vi "TEST_L0_SUM_(1ST).vi"(4 "Voltages comprobation":dbl[](array[numeric])=[0.05, 0.1, 0.2, 0.5, 0.8], 5 "Serial number":string="SN018", 6 "IB_Clip":i32[](array[numeric])=[7, 23, 31, 63], 7 "Save NOW!":bool, 8 "error in":errorcluster, 9 "Cycles Burst":i32=10000, 10 "Channels":i32[](array[numeric])=[0, 1, 2, 3, 4, 5, 6], 11 "Instrument VISA in":T1={"AWG VISA"="generadorpulsos", "Oscilloscope  VISA "="Oscilloscope", "Integration Board IP"="172.16.7.43", "connection ID"=refnum, "report out"=refnum, "report file path"=path "C:/Documents and Settings/CTA_LAB01/Desktop/L0_Asic/L0 Asic Test Data"}) -> (0 "error out":errorcluster, 3 "Instrument VISA out":T1={"AWG VISA"="generadorpulsos", "Oscilloscope  VISA "="Oscilloscope", "Integration Board IP"="172.16.7.43", "connection ID"=refnum, "report out"=refnum, "report file path"=path "C:/Documents and Settings/CTA_LAB01/Desktop/L0_Asic/L0 Asic Test Data"})   [LabVIEW 2009]
uses:
  <vilib>/Utility/NIReport.llb/NI_report.lvclass
  <vilib>/Utility/NIReport.llb/HTML/NI_HTML.lvclass
  Sum_Abrilader/L0_Sum_Adder Folder/C/Program Files/National Instruments/LabVIEW 2012/instr.lib/Agilent 8000 Series/Public/Configure/Configure Math (Binary Operation).vi
  <instrlib>/Agilent 8000 Series/Public/Data/Read (Multiple Waveforms).vi
  Sum_Abrilader/L0_Sum_Adder Folder/C/Program Files/National Instruments/LabVIEW 2012/instr.lib/Agilent 81150/Agilent 81150.lvlib
  Sum_Abrilader/L0_Sum_Adder Folder/C/Program Files/National Instruments/LabVIEW 2012/instr.lib/Agilent 8000 Series/Agilent 8000 Series.lvlib
panel:
  out "ClipRect":dbl=136149.0
  in  "Atenuation":i32[](array[numeric])=[0, 15]
  out "dt":dbl=3.125e-12
  out "report file path":path=path "C:/Documents and Settings/CTA_LAB01/Desktop/L0_Asic/L0 Asic Test Data"
  in  "Full waveform":bool
  out "Waveform Data":waveform(dbl)[](graph)=[{"t0"=timestamp(-6.010937525502413e-09 s since 1904-01-01), "dt"=3.125e-12, "Y"=array[6408 elements]}, {"t0"=timestamp(-6.010937525502413e-09 s since 1904-01-01), "dt"=3.125e-12, "Y"=array[6408 elements]}]
  out "time for channel bucle":u32=4294966675
  out "iindex inner bucle":u16=109
  out "time attenuation bucle":u32=136149
  out "points quantity":dbl=15.0
  out "appended array":dbl[](array[numeric])=[9.99999e+37, 9.99999e+37, 2.137332e-09, 7.2166e-11, 9.99999e+37, 9.99999e+37, 9.99999e+37, 9.99999e+37, 9.99999e+37, 9.99999e+37, 15.0]
  out "read buffer 3":string="V amptd(1),9.99999E+37,9.99999E+37,9.99999E+37,9.99999E+37,9.99999E+37,1.5E+01,+ width(1),2.18163E-09,2.01279E-09,2.26658E-09,2.137332E-09,7.2166E-11,1.5E+01,V amptd(f2),9.99999E+37,9.99999E+37,9.99999E+37,9.99999E+37,9.99999E+37,1.5E+01,+ width(f2),9.99999E+37,9.99999E+37,9.99999E+37,9.99999E+37,9.99999E+37,9E+00,Time(1-f2),9.99999E+37,9.99999E+37,9.99999E+37,9.99999E+37,9.99999E+37,1.3E+01\n"
  out "bucle for inner bucle":u32=363
  out "Numeric":i32=9300975
  in  "Clip_sel_b":u32
  in  "Att gain":u32=4095
  in  "Quantity of measurements":u32=50
  in  "End 2":bool
  out "Data output":dbl[][](array[numeric])=[[0.05, 0.0, 15.0, 7.0, 1.0, 9.99999e+37, 9.99999e+37, 2.14249e-09, 8.3497e-11, 9.99999e+37, 9.99999e+37, 9.99999e+37, 9.99999e+37, 9.99999e+37, 9.99999e+37, 17.0, 0.0336, -0.00019404761904761897, 105.0], [0.05, 0.0, 15.0, 31.0, 1.0, 9.99999e+37, 9.99999e+37, 2.188109e-09, 8.187e-11, 9.99999e+37, 9.99999e+37, 9.99999e+37, 9.99999e+37, 9.99999e+37, 9.99999e+37, 14.0, 0.0336, -0.00019404761904761897, 106.0], [0.05, 0.0, 15.0, 63.0, 1.0, 9.99999e+37, 9.99999e+37, 2.133683e-09, 8.8016e-11, 9.99999e+37, 9.99999e+37, 9.99999e+37, 9.99999e+37, 9.99999e+37, 9.99999e+37, 15.0, 0.0336, -0.00019404761904761897, 107.0], [0.05, 1.0, 15.0, 7.0, 1.0, 9.99999e+37, 9.99999e+37, 2.137332e-09, 7.2166e-11, 9.99999e+37, 9.99999e+37, 9.99999e+37, 9.99999e+37, 9.99999e+37, 9.99999e+37, 15.0, 0.0336, -0.00019404761904761897, 108.0]]
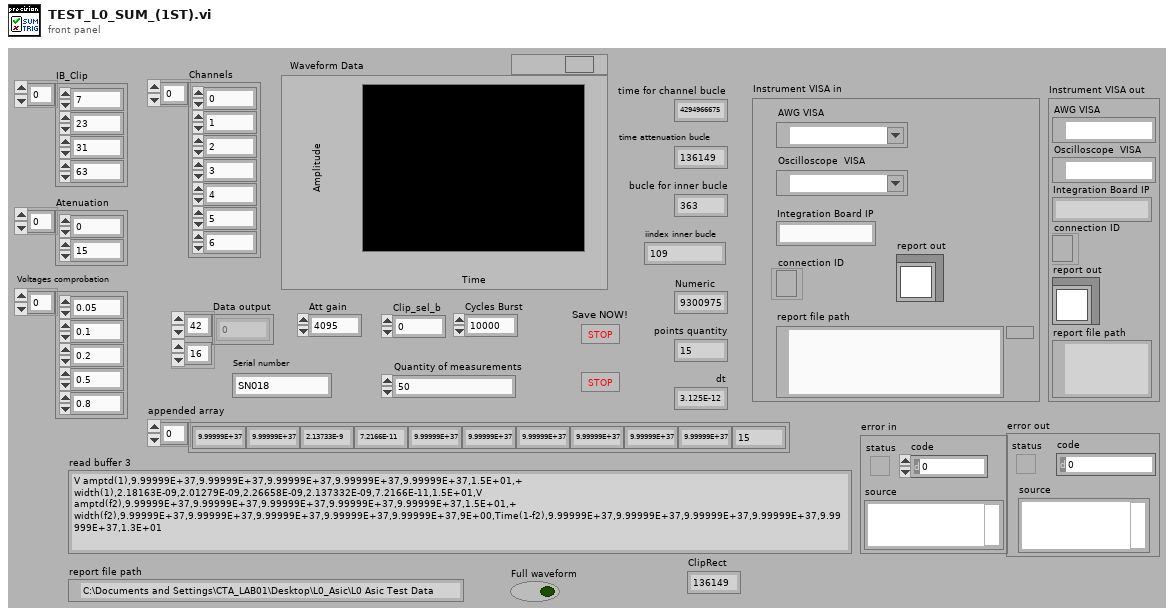
[diagram p1: front panel]
types:
  T1 = cluster{"AWG VISA":refnum<visa-resource-name>, "Oscilloscope  VISA ":refnum<visa-resource-name>, "Integration Board IP":string, "connection ID":refnum<k5>, "report out":refnum<class "NI_report.lvclass">, "report file path":path}
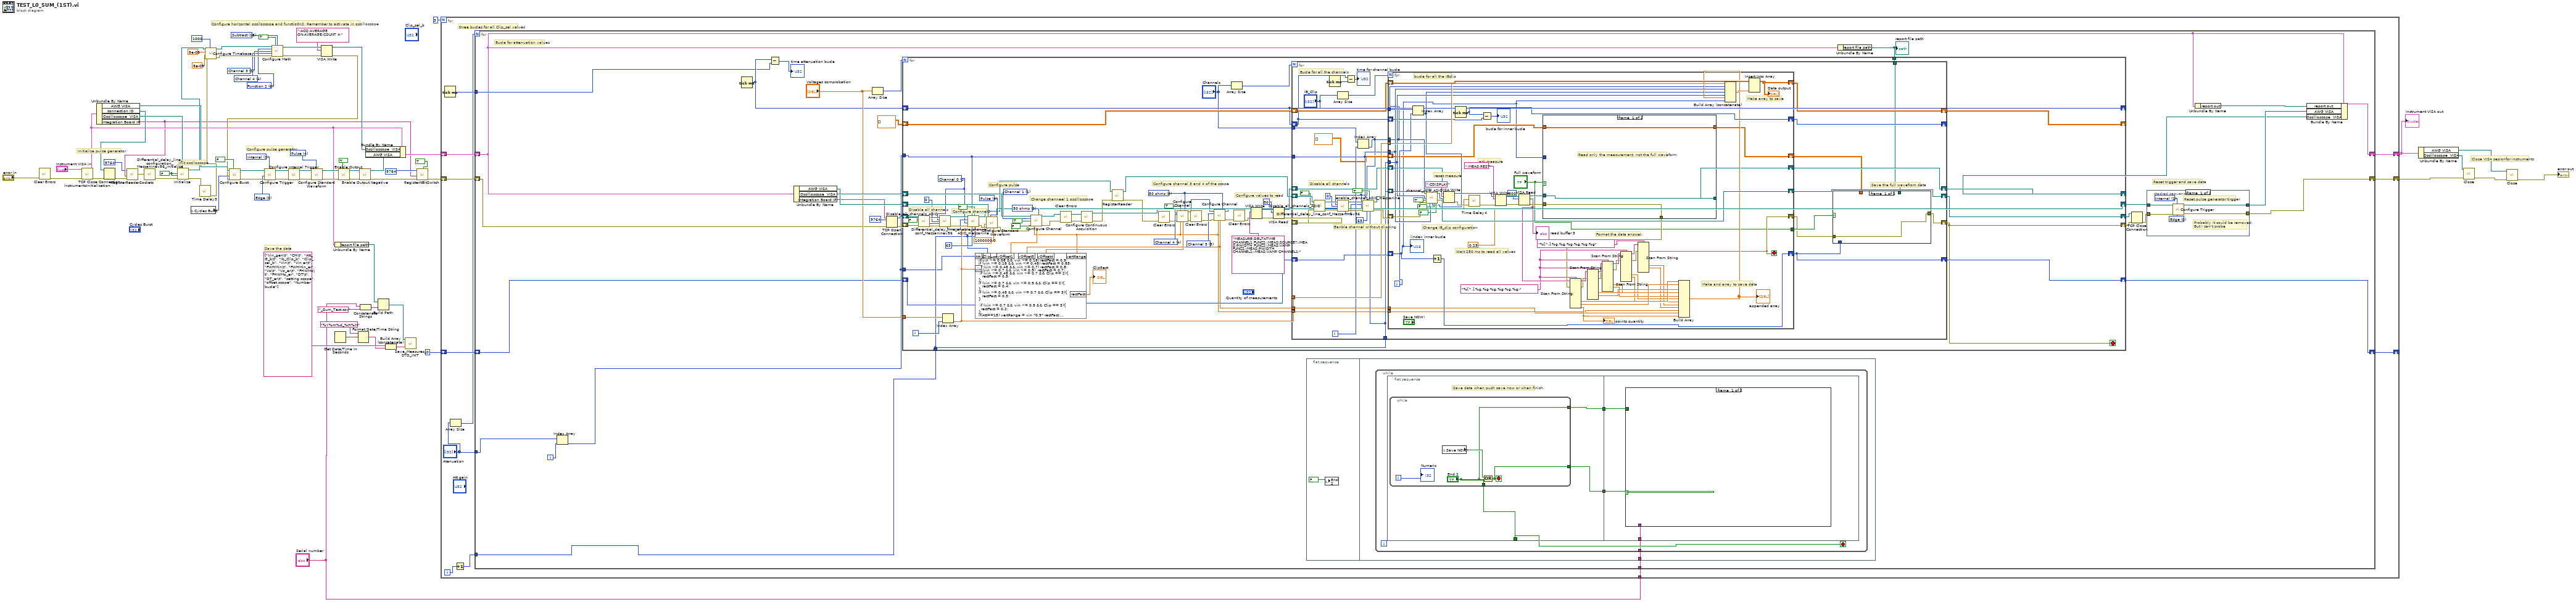
[diagram p0: block diagram]
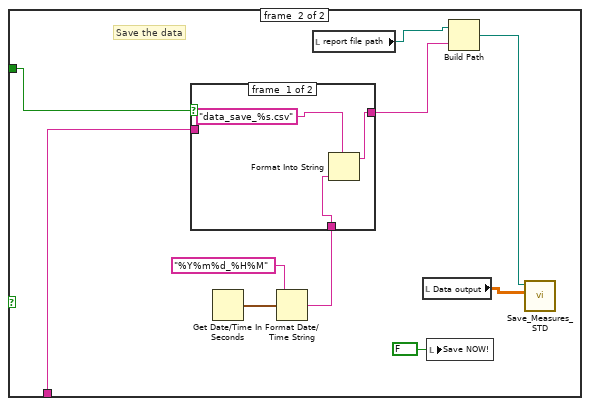
[diagram p2: hidden frame]
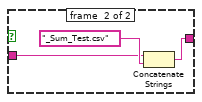
[diagram p3: hidden frame]
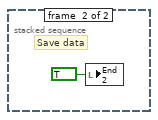
[diagram p4: hidden frame]
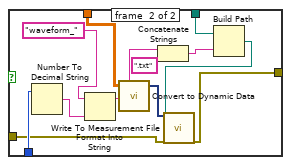
[diagram p5: hidden frame]
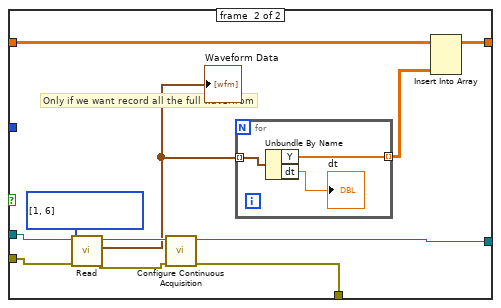
[diagram p6: hidden frame]
diagram:
  w44 = u16 6 items=["Function 1"=5, "Function 2"=6, "Function 3"=7, "Function 4"=8] ("Math Channel (5: Function 1)")
  w48 = u16 15 items=["Add"=12, "Divide"=13, "Multiply"=14, "Subtract"=15, "Common Mode"=16, "Versus"=17] ("Math Operation (12: Add)")
  w43 = 3 items=["Channel 1"=1, "Channel 2"=2, "Channel 3"=3, "Channel 4"=4] ("Channel (1: Channel 1)")
  w42 = 4 items=["Channel 1"=1, "Channel 2"=2, "Channel 3"=3, "Channel 4"=4] ("Channel (1: Channel 1)")
  w63 = u16 1 items=["Immediate", "Internal", "External", "Software Trigger Function"] ("Trigger Source (0: Immediate)")
  w64 = u16 0 items=["Edge", "Level"] ("Trigger Mode (0: Edge)")
  w68 = u16 4 items=["Sine", "Square", "Ramp Up", "Ramp Down", "Pulse", "Noise", "DC"] ("Waveform (0: Sine)")
  w72 = FALSE ("ID Query (True)")
  # "Save the data"
  # "Configure horizontal osciloscope and functio0n2. Remember to activate in oscilloscope"
  # "Close VISA sesionfor instruments"
  # "Configure pulse generator"
  # "Init osciloscope"
  # "Initialize pulse generator"
  n1 = call <vilib>:"Clear Errors.vi"("error in (no error)"="error in") -> ("error out"=w70:errorcluster)  [unwired: 6 in]
  n2 = call "instrumentsInitialization.vi"("error in"=w70, "Instrument VISA in"="Instrument VISA in") -> ("error out"=w11:errorcluster, "Instrument VISA out"=w19:T1)  [unwired: 8 in]
  n3 = Unbundle By Name(w19) -> ("AWG VISA"=w54:refnum<visa-resource-name>, "connection ID"=w58:refnum<k5>, "Oscilloscope  VISA"=w55:refnum<visa-resource-name>, "Integration Board IP"=w3:string)
  n4 = TCP Close Connection(connection ID=w58, error in (no error)=w11) -> (error out=w4:errorcluster)  [unwired: 1 in, 1 out]
  n5 = call "RegisterReaderSockets.vi"("error in (no error)"=w4, "IP"=w3, "Port"=u16 9764 ("remote port or service name")) -> ("error out"=w1:errorcluster)  [unwired: 7 in]
  n6 = call "Differential_delay_line_configuration_Mezzaninev56_initialize.vi"("error in (no error)"=w1) -> ("error out 2"=w10:errorcluster)  [unwired: 1 in]
  n7 = call "Initialize.vi"("error in (no error)"=w10, "Reset (True)"=w72, "ID Query (True)"=w72, "VISA resource name"=w55) -> ("error out"=w71:errorcluster, "VISA resource name out"=w41:refnum<visa-resource-name>)  [unwired: 6 in]
  n8 = local read "Cycles Burst"() -> (w67:i32)
  n9 = call "Time Delay3"("error in (no error)"=w71) -> ("error out"=w40:errorcluster)  [unwired: 10 in]
  n10 = call "Configure Timebase.vi"("Record Length (1000)"=1000, "error in (no error)"=w40, "Position (0.0 s)"=8e-09, "Timebase (0.005 s)"=5e-08, "VISA resource name"=w41) -> ("error out"=w45:errorcluster, "VISA resource name out"=w46:refnum<visa-resource-name>)  [unwired: 5 in]
  n11 = call-poly "Configure Math.vi"("VISA resource name"=w46, "Enable Math Channel (T:Enable)"=TRUE, "Math Operation (12: Add)"=w48, "Math Channel (5: Function 1)"=w44, "Math Operand (1: Channel 1)"=w43, "Math Operand (2: Channel 2)"=w42, "error in (no error)"=w45) -> ("VISA resource name out"=w16:refnum<visa-resource-name>, "error out"=w15:errorcluster)  [unwired: 7 in]
  n12 = VISA Write(VISA resource name=w16, write buffer=":ACQ:AVERAGE ON;AVERAGE:COUNT 4;", error in (no error)=w15) -> (VISA resource name out=w13:refnum<visa-resource-name>, error out=w14:errorcluster)  [unwired: 1 out]
  n13 = call "Configure Burst.vi"("Enable Burst (F: Disable)"=FALSE, "error in (no error)"=w14, "Burst Count (2)"=w67, "VISA resource name"=w54) -> ("error out"=w66:errorcluster, "VISA resource name out"=w65:refnum<visa-resource-name>)  [unwired: 6 in]
  n14 = call "Configure Trigger.vi"("Trigger Source (0: Immediate)"=w63, "error in (no error)"=w66, "Trigger Mode (0: Edge)"=w64, "VISA resource name"=w65) -> ("error out"=w62:errorcluster, "VISA resource name out"=w61:refnum<visa-resource-name>)  [unwired: 6 in]
  n15 = call "Configure Internal Trigger.vi"("error in (no error)"=w62, "VISA resource name"=w61) -> ("error out"=w59:errorcluster, "VISA resource name out"=w60:refnum<visa-resource-name>)  [unwired: 8 in]
  n16 = call "Configure Standard Waveform.vi"("Waveform (0: Sine)"=w68, "error in (no error)"=w59, "VISA resource name"=w60) -> ("error out"=w53:errorcluster, "VISA resource name out"=w52:refnum<visa-resource-name>)  [unwired: 7 in]
  n17 = Unbundle By Name(w19) -> ("report file path"=w20:path)
  n18 = Get Date/Time In Seconds() -> (seconds since 1Jan1904=w25:timestamp)
  n19 = call "Enable Output.vi"("Enable Output (T: Enable)"=TRUE, "error in (no error)"=w53, "VISA resource name"=w52) -> ("error out"=w31:errorcluster, "VISA resource name out"=w30:refnum<visa-resource-name>)  [unwired: 7 in]
  n20 = Format Date/Time String(time format string (%c)="%Y%m%d_%H%M", seconds (now)=w25) -> (date/time string=w23:string)  [unwired: 1 in]
  n21 = call "Enable Output Negative.vi"("error in (no error)"=w31, "VISA resource name"=w30) -> ("error out"=w9:errorcluster, "VISA resource name out"=w29:refnum<visa-resource-name>)  [unwired: 8 in]
  n22 = Concatenate Strings("Serial number", "_Sum_Test.csv" ("format string")) -> (w21:string)
  n23 = Bundle By Name(cluster=w19, "Oscilloscope  VISA"=w13, "AWG VISA"=w29) -> (w7:T1)
  n24 = Build Path(base path=w20, name or relative path=w21) -> (appended path=w28:path)
  n25 = Build Array (concatenate)(string[] ["Vin_gen\t", "CH\t", "Att_G_b\t", "Ib_Clip_b", "Clip_sel_b", "Vin\t", "Vin er\t", "FWHMin\t", "FWHMin_er", "Vo\t", "Vo_er\t", "FHWMo\t", "FHWMo_er", "DT\t", "DT_er\t", "setting scope", "offset scope", "Number bucle"] ("appended array"), w23) -> (w26:string[])
  n26 = call "Save_Measures_STD_INIT.vi"("appended array"=w26, "file path (dialog if empty)"=w28) -> ()  [unwired: 10 in]
  n27 = call "RegisterNBitSwitch.vi"("Switch Bit"=TRUE ("Enable Output (T: Enable)"), "error in (no error)"=w9, "IP"=w3, "Port"=u16 9764 ("remote port or service name")) -> ("error out"=w8:errorcluster)  [unwired: 7 in]
  n28 = for {
    N: 3 -> [_]
    shift-right: [w84] -> w35
    shift-left: w8 -> [w80]
    shift-right: [w83] -> w18
    shift-left: w7 -> [w79]
    shift-right: [w76] -> _
    shift-left: u16 0 ("remote port or service name") -> [w77]
    tunnel: "Serial number" -> [w73]
    i -> [w81]
    # "three bucles for all Clip_sel values"
    n29 = Tick Count (ms)() -> (millisecond timer value=w78:u32)
    n30 = Array Size(array="Atenuation") -> (size(s)=w75:i32)
    n31 = Increment(x=w81) -> (x+1=w82:i32)
    n32 = for {
      N: w75 -> [_]
      shift-right: [w89] -> w84
      shift-left: w80 -> [w106]
      shift-right: [w113] -> w83
      shift-left: w79 -> [w93]
      tunnel: w82 -> [w91]
      tunnel: w78 -> [w98]
      shift-right: [w96] -> w76
      shift-left: w77 -> [w97]
      tunnel: "Atenuation" -> [w87]
      tunnel: w73 -> [w86]
      i -> [w88]
      # "Reset trigger and save data"
      # "Bucle for attenuation values"
      n33 = Index Array(array=w87, index=w88) -> (element=w85:i32)
      n34 = Tick Count (ms)() -> (millisecond timer value=w99:u32)
      n35 = Subtract(x=w99, y=w98) -> (x-y=→"time attenuation bucle":u32)
      n36 = Unbundle By Name(w93) -> ("AWG VISA"=w110:refnum<visa-resource-name>, "Oscilloscope  VISA"=w111:refnum<visa-resource-name>, "Integration Board IP"=w107:string)
      n37 = Array Size(array="Voltages comprobation") -> (size(s)=w114:i32)
      n38 = TCP Open Connection(address=w107, remote port or service name=u16 9764, error in (no error)=w106) -> (connection ID=w101:refnum<k5>, error out=w105:errorcluster)  [unwired: 2 in]
      n39 = flat-sequence {
        tunnel: w86 -> [w117]
        frame #0 {
          n40 = local write "End 2"(FALSE ("End")) -> ()
        }
        frame #1 {
          n41 = while {
            tunnel: w117 -> [w118]
            stop <- w119 stop-if-true
            n42 = flat-sequence {
              tunnel: [w124] -> w121
              tunnel: [w123] -> w120
              tunnel: [w122] -> w119
              tunnel: w121 -> [w131]
              tunnel: w120 -> [w130]
              tunnel: w118 -> [w129]
              frame #0 {
                # "Save data when push save now or when finish."
                n43 = while {
                  tunnel: [w127] -> w124
                  tunnel: ["End 2"] -> w123
                  tunnel: ["End 2"] -> w122
                  i -> [w126]
                  stop <- w127 stop-if-true
                  n44 = local read "Save NOW!"() -> (w128:bool)
                  n45 = Or(x=w128, y="End 2") -> (x .or. y?=w127:bool)
                  "Numeric" <- w126
                }
              }
              frame #1 {
                n46 = case shown="True" w131 {
                  tunnel: w130 -> [_ w138]
                  tunnel: w129 -> [_ w132]
                  frame #0 {
                  }
                  frame #1 {
                    # "Save the data"
                    n47 = Get Date/Time In Seconds() -> (seconds since 1Jan1904=w135:timestamp)
                    n48 = Format Date/Time String(time format string (%c)="%Y%m%d_%H%M", seconds (now)=w135) -> (date/time string=w133:string)  [unwired: 1 in]
                    n49 = case shown="True" w138 {
                      tunnel: [w143 w145] -> w137
                      tunnel: w133 -> [w142 _]
                      tunnel: w132 -> [_ w146]
                      frame #0 {
                        n50 = Format Into String(format string="data_save_%s.csv", w142) -> (resulting string=w143:string)  [unwired: 2 in, 1 out]
                      }
                      frame #1 {
                        n51 = Concatenate Strings(w146, "_Sum_Test.csv" ("format string")) -> (w145:string)
                      }
                    }
                    n52 = local read "report file path"() -> (w136:path)
                    n53 = local read "Data output"() -> (w140:dbl[][])
                    n54 = local write "Save NOW!"(FALSE ("Save NOW!")) -> ()
                    n55 = Build Path(base path=w136, name or relative path=w137) -> (appended path=w141:path)
                    n56 = call "Save_Measures_STD.vi"("Data in"=w140, "file path (dialog if empty)"=w141) -> ()  [unwired: 10 in]
                  }
                }
              }
            }
          }
        }
      }
      n57 = Unbundle By Name(w93) -> ("report file path"=w92:path)
      "report file path" <- w92
      n58 = for {
        N: w114 -> [_]
        shift-right: [w159] -> w103
        shift-left: w105 -> [w203]
        shift-right: [w216] -> _
        shift-left: dbl[][] [] -> [w217]
        tunnel: "Voltages comprobation" -> [w215]
        shift-right: [w195] -> w112
        shift-left: w110 -> [w223]
        shift-right: [w212] -> w94
        shift-left: w111 -> [w208]
        tunnel: w85 -> [w210]
        tunnel: w91 -> [w173]
        shift-right: [w160] -> w102
        shift-left: w101 -> [w202]
        shift-right: [w180] -> _
        shift-left: w99 -> [w180]
        shift-right: [w179] -> w96
        shift-left: w97 -> [w191]
        tunnel: w92 -> [w178]
        tunnel: w85 -> [w172]
        i -> [w222]
        stop <- w159 stop-if-true
        w184 = 3 items=["Channel 1"=1, "Channel 2"=2, "Channel 3"=3, "Channel 4"=4] ("Channel (1: Channel 1)")
        w204 = 4 items=["Channel 1"=1, "Channel 2"=2, "Channel 3"=3, "Channel 4"=4] ("Channel (1: Channel 1)")
        w185 = u32 0 items=["50 ohms", "1 Mohms"] ("Input Impedance (1: 1 Mohms)")
        w162 = u16 0 items=["Channel 0", "Channel 1", "Channel 2", "Channel 3", "Channel 4", "Channel 5", "Channel 6"] ("Channel")
        w219 = u32 0 items=["50 ohms", "1 Mohms"] ("Input Impedance (1: 1 Mohms)")
        w221 = 1 items=["Channel 1"=1, "Channel 2"=2, "Channel 3"=3, "Channel 4"=4] ("Channel (1: Channel 1)")
        w224 = u16 4 items=["Sine", "Square", "Ramp Up", "Ramp Down", "Pulse", "Noise", "DC"] ("Waveform (0: Sine)")
        # "Configure values to read"
        # "Configure channel 3 and 4 of the scope"
        # "Change channeel 1 oscilloscope"
        # "Configure pulse"
        # "Configure channel0"
        # "Disable all channels"
        n59 = call "Disable_all_channels_ASIC.vi"("error in"=w203, "Clip_en_b"=FALSE, "connection ID"=w202) -> ("error out"=w168:errorcluster, "id_out"=w163:i32, "connection ID out"=w164:refnum<k5>)  [unwired: 6 in]
        n60 = call "Differential_delay_line_conf_Mezzaninev56.vi"("connection ID"=w164, "channel"=w162, "Delay value"=u16 0, "Id in"=w163, "error in (no error)"=w168) -> ("connection ID out"=w165:refnum<k5>, "Id out"=w166:i32, "error out 2"=w167:errorcluster)  [unwired: 3 in, 5 out]
        n61 = Index Array(array=w215, index=w222) -> (element=w174:dbl)
        n62 = call "enable_channel_ASIC_mezzanine.vi"("Clip_sel_b"=w173, "maj/sum"=TRUE, "Ib_clipVb"=u32 63, "Att gain"=w210, "error in"=w167, "Channel"=w162, "id_in"=w166, "connection ID"=w165) -> ("error out"=w211:errorcluster, "connection ID out"=w156:refnum<k5>)  [unwired: 1 in, 1 out]
        n63 = formula code="float rectFact = 1;\nif(vin >= 0.08 && vin <= 0.18) rectFact = 0.9;\nif (vin >= 0.18 && vin <= 0.48) rectFact = 0.85;\n if (vin >= 0.48 && vin <= 0.7) rectFact = 0.8;\nif (vin >= 0.7 && vin <= 0.9)  rectFact = 0.7;\n if (vin >= 0.48 && vin <= 0.7 && Clip == 2){\n   rectFact = 0.5;\n}\nif (vin >= 0.7 && vin <= 0.9 && Clip == 2){\n   rectFact = 0.4;\n}\nif (vin >= 0.48 && vin <= 0.7 && Clip == 3){\n   rectFact = 0.3;\n}\n\n if (vin >= 0.7 && vin <= 0.9 && Clip == 3){\n  rectFact = 0.2;\n}\nif(Att==15) vertRange = vin *0.9* rectFact;\nelse vertRange = vin * 1.0* rectFact;\nvOffset1  = vertRange /6;\nvOffset3  = vertRange /6;\nvOffset4  = -vertRange/6;"("vin"=w174, "Att"=w172, "Clip"=w173) -> ("vOffset1"=w176:dbl, "vOffset3"=w169:dbl, "vOffset4"=w175:dbl, "vertRange"=w170:dbl, "rectFact"=→"ClipRect":dbl)
        n64 = call "Configure Standard Waveform.vi"("Frequency (1000.0 Hz)"=1000000.0, "Waveform (0: Sine)"=w224, "error in (no error)"=w211, "Amplitude (1.0 Vpp)"=w174, "VISA resource name"=w223) -> ("error out"=w209:errorcluster, "VISA resource name out"=w195:refnum<visa-resource-name>)  [unwired: 5 in]
        n65 = call "Configure Channel.vi"("VISA resource name"=w208, "Enable Channel (Enable)"=TRUE, "BW Limit 20MHz (Disable)"=FALSE, "Input Impedance (1: 1 Mohms)"=w219, "Channel (1: Channel 1)"=w221, "error in (no error)"=w209, "Vertical Range (2.0 V)"=w170, "Vertical Offset (0.0 V)"=w176) -> ("VISA resource name out"=w207:refnum<visa-resource-name>, "error out"=w206:errorcluster)  [unwired: 6 in]
        n66 = call <vilib>:"Clear Errors.vi"("error in (no error)"=w206) -> ("error out"=w205:errorcluster)  [unwired: 6 in]
        n67 = call "Configure Continuous Acquisition.vi"("error in (no error)"=w205, "VISA resource name"=w207) -> ("error out"=w158:errorcluster, "VISA resource name out"=w177:refnum<visa-resource-name>)  [unwired: 8 in]
        n68 = call "RegisterReader.vi"("error in (no error)"=w158, "connection ID"=w156) -> ("error out"=w157:errorcluster, "connection ID out"=w155:refnum<k5>)  [unwired: 7 in]
        n69 = call <vilib>:"Clear Errors.vi"("error in (no error)"=w157) -> ("error out"=w213:errorcluster)  [unwired: 6 in]
        n70 = call "Configure Channel.vi"("VISA resource name"=w177, "Enable Channel (Enable)"=TRUE, "Input Impedance (1: 1 Mohms)"=w185, "Channel (1: Channel 1)"=w204, "error in (no error)"=w213, "Vertical Range (2.0 V)"=w170, "Vertical Offset (0.0 V)"=w175) -> ("VISA resource name out"=w187:refnum<visa-resource-name>, "error out"=w214:errorcluster)  [unwired: 7 in]
        n71 = call <vilib>:"Clear Errors.vi"("error in (no error)"=w214) -> ("error out"=w189:errorcluster)  [unwired: 6 in]
        n72 = call "Configure Channel.vi"("VISA resource name"=w187, "Input Impedance (1: 1 Mohms)"=w185, "Channel (1: Channel 1)"=w184, "error in (no error)"=w189, "Vertical Range (2.0 V)"=w170, "Vertical Offset (0.0 V)"=w169) -> ("VISA resource name out"=w186:refnum<visa-resource-name>, "error out"=w190:errorcluster)  [unwired: 8 in]
        n73 = Array Size(array="Channels") -> (size(s)=w196:i32)
        n74 = call <vilib>:"Clear Errors.vi"("error in (no error)"=w190) -> ("error out"=w188:errorcluster)  [unwired: 6 in]
        n75 = VISA Write(VISA resource name=w186, write buffer="MEASURE:DELTATIME CHANNEL1,FUNC2;:MEAS:SOURCE?;:MEAS:PWIDTH FUNC2;:MEAS:VAMP FUNC2;:MEAS:PWIDTH CHANNEL1;:MEAS:VAMP CHANNEL1;", error in (no error)=w188) -> (VISA resource name out=w201:refnum<visa-resource-name>, error out=w200:errorcluster)  [unwired: 1 out]
        n76 = VISA Read(VISA resource name=w201, byte count=u32 50, error in (no error)=w200) -> (VISA resource name out=w197:refnum<visa-resource-name>, error out=w198:errorcluster)  [unwired: 2 out]
        n77 = for {
          N: w196 -> [_]
          tunnel: w210 -> [w243]
          tunnel: w173 -> [w251]
          tunnel: w174 -> [w263]
          shift-right: [w265] -> w216
          shift-left: w217 -> [w266]
          shift-right: [w264] -> w212
          shift-left: w197 -> [w261]
          shift-right: [w262] -> w160
          shift-left: w155 -> [w255]
          shift-right: [w241] -> w159
          shift-left: w198 -> [w257]
          tunnel: "Channels" -> [w260]
          shift-right: [w237] -> w179
          shift-left: w191 -> [w258]
          shift-right: [w245] -> _
          shift-left: w180 -> [w246]
          tunnel: w178 -> [w239]
          tunnel: w170 -> [w235]
          tunnel: w169 -> [w234]
          i -> [w259]
          # "Eanble channel without clipping"
          # "Disable all channels"
          # "Save the full wavefrom data"
          # "Bucle for all the channels"
          n78 = call "Disable_all_channels_ASIC.vi"("error in"=w257, "Clip_en_b"=FALSE, "connection ID"=w255) -> ("error out"=w233:errorcluster, "id_out"=w229:i32, "connection ID out"=w231:refnum<k5>)  [unwired: 6 in]
          n79 = Tick Count (ms)() -> (millisecond timer value=w247:u32)
          n80 = Array Size(array="IB_Clip") -> (size(s)=w249:i32)
          n81 = Subtract(x=w246, y=w247) -> (x-y=→"time for channel bucle":u32)
          n82 = Index Array(array=w260, index=w259) -> (element=w228:i32)
          n83 = call "Differential_delay_line_conf_Mezzaninev56.vi"("connection ID"=w231, "channel"=w228, "Delay value"=u16 0, "Id in"=w229, "error in (no error)"=w233) -> ("connection ID out"=w230:refnum<k5>, "Id out"=w227:i32, "error out 2"=w232:errorcluster)  [unwired: 3 in, 5 out]
          n84 = call "enable_channel_ASIC_mezzanine.vi"("Clip_sel_b"=w251, "maj/sum"=TRUE, "Ib_clipVb"=u32 63, "Att gain"=w243, "error in"=w232, "Channel"=w228, "id_in"=w227, "connection ID"=w230) -> ("error out"=w256:errorcluster, "connection ID out"=w254:refnum<k5>)  [unwired: 1 in, 1 out]
          n85 = for {
            N: w249 -> [_]
            shift-right: [w289] -> w240
            shift-left: w256 -> [w313]
            tunnel: w263 -> [w344]
            shift-right: [w326] -> w265
            shift-left: w266 -> [w342]
            tunnel: w243 -> [w339]
            shift-right: [w291] -> w264
            shift-left: w261 -> [w315]
            tunnel: w251 -> [w338]
            shift-right: [w340] -> w262
            shift-left: w254 -> [w341]
            shift-right: [w335] -> w245
            shift-left: w246 -> [w336]
            tunnel: w228 -> [w298]
            shift-right: [w297] -> w237
            shift-left: w258 -> [w284]
            tunnel: "IB_Clip" -> [w296]
            shift-right: [w287] -> w238
            shift-left: dbl[][] [] ("Y") -> [w288]
            tunnel: ["Full waveform"] -> w242
            tunnel: w235 -> [w282]
            tunnel: w234 -> [w281]
            i -> [w295]
            stop <- w289 stop-if-true
            w308 = "%[^,],%g,%g,%g,%g,%g,%g," ("format string")
            # "Make and array to save data"
            # "Wait 250 ms to read all values"
            # "Change IB_clip configuration"
            # "Make array to save"
            # "Format the data answer."
            # "ask measure"
            # "reset measure"
            # "bucle for all the IBclip"
            n86 = Index Array(array=w296, index=w295) -> (element=w294:i32)
            n87 = call "channel_conf_ASIC.vi"("connection ID"=w341, "Ring"=w298, "Clip_sel_b"=w338, "CompBuf_en_b"=TRUE, "error out"=w313, "Att gain"=w339, "Ib_ClipVb"=w294, "Clip_en_b"=FALSE, "Att_en_b"=FALSE) -> ("connection ID out"=w340:refnum<k5>, "error out 2"=w311:errorcluster)  [unwired: 2 in, 3 out]
            n88 = Increment(x=w284) -> (x+1=w297:u16)
            n89 = VISA Write(VISA resource name=w315, write buffer=":CDISPLAY", error in (no error)=w311) -> (VISA resource name out=w317:refnum<visa-resource-name>, error out=w310:errorcluster)  [unwired: 1 out]
            n90 = Tick Count (ms)() -> (millisecond timer value=w335:u32)
            n91 = call "Time Delay4"("error in (no error)"=w310, "Delay Time (s)"=0.25 ("x*y")) -> ("error out"=w328:errorcluster)  [unwired: 9 in]
            n92 = Subtract(x=w335, y=w336) -> (x-y=→"bucle for inner bucle":u32)
            n93 = VISA Write(VISA resource name=w317, write buffer=":MEAS:RES?", error in (no error)=w328) -> (VISA resource name out=w333:refnum<visa-resource-name>, error out=w332:errorcluster)  [unwired: 1 out]
            n94 = VISA Read(VISA resource name=w333, byte count=u32 800, error in (no error)=w332) -> (VISA resource name out=w292:refnum<visa-resource-name>, read buffer=w329:string, error out=w293:errorcluster)  [unwired: 1 out]
            "read buffer 3" <- w329
            n95 = case shown="False" "Full waveform" {
              tunnel: w293 -> [w347 w356]
              tunnel: w292 -> [w346 w358]
              tunnel: [w346 w354] -> w291
              tunnel: [w347 w348] -> w290
              tunnel: w284 -> [_ _]
              tunnel: w288 -> [w345 w351]
              tunnel: [w345 w350] -> w287
              frame #0 {
                # "Read only the measurement, not the full waveform"
              }
              frame #1 {
                w357 = i32[] [1, 6] items=["Channel 1"=1, "Channel 2"=2, "Channel 3"=3, "Channel 4"=4, "Function 1"=5, "Function 2"=6, "Function 3"=7, "Function 4"=8, "Memory 1"=9, "Memory 2"=10, "Memory 3"=11, "Memory 4"=12] ("Channels")
                # "Only if we want record all the full waverfrom"
                n96 = call-poly <instrlib>:"Read.vi"("error in (no error)"=w356, "Channels"=w357, "VISA resource name"=w358) -> ("error out"=w353:errorcluster, "Waveform Data"=w352:waveform(dbl)[], "VISA resource name out"=w355:refnum<visa-resource-name>)  [unwired: 6 in]
                "Waveform Data" <- w352
                n97 = call "Configure Continuous Acquisition.vi"("error in (no error)"=w353, "VISA resource name"=w355) -> ("error out"=w348:errorcluster, "VISA resource name out"=w354:refnum<visa-resource-name>)  [unwired: 8 in]
                n98 = for {
                  tunnel: w352 -> [w361] mode=indexing
                  tunnel: [w360] -> w349 mode=indexing
                  n99 = Unbundle By Name(w361) -> ("Y"=w360:dbl[], "dt"=→"dt":dbl)
                }
                n100 = Insert Into Array(array=w351, new element=w349) -> (w350:dbl[][])  [unwired: 2 in]
              }
            }
            n101 = Scan From String(format string=w308, input string=w329, error in=w290) -> (remaining string=w325:string, error out=w318:errorcluster, output 5=w307:dbl, output 6=w306:dbl, output 7=w283:dbl)  [unwired: 12 in, 1 out]
            "points quantity" <- w283
            n102 = Scan From String(format string=w308, input string=w325, error in=w318) -> (remaining string=w322:string, error out=w319:errorcluster, output 5=w305:dbl, output 6=w304:dbl)  [unwired: 13 in, 1 out]
            n103 = Scan From String(format string=w308, input string=w322, error in=w319) -> (remaining string=w323:string, error out=w320:errorcluster, output 5=w280:dbl, output 6=w303:dbl)  [unwired: 13 in, 1 out]
            n104 = Scan From String(format string=w308, input string=w323, error in=w320) -> (remaining string=w324:string, error out=w321:errorcluster, output 5=w302:dbl, output 6=w301:dbl)  [unwired: 13 in, 1 out]
            n105 = Scan From String(format string="%[^,],%g,%g,%g,%g,%g,%g", input string=w324, error in=w321) -> (error out=w289:errorcluster, output 5=w300:dbl, output 6=w299:dbl)  [unwired: 13 in, 2 out]
            n106 = Build Array(w307, w306, w305, w304, w280, w303, w302, w301, w300, w299, w282, w281, w283) -> (w327:dbl[])
            "appended array" <- w327
            n107 = Build Array (concatenate)(w344, w298, w339, w294, w338, w327, w284) -> (w343:dbl[])
            n108 = Insert Into Array(array=w342, new element=w343) -> (w326:dbl[][])  [unwired: 2 in]
            "Data output" <- w326
            "iindex inner bucle" <- w284
          }
          n109 = case shown="False" w242 {
            tunnel: w238 -> [_ w279]
            tunnel: w240 -> [w267 w268]
            tunnel: [w267 w277] -> w241
            tunnel: w239 -> [_ w270]
            tunnel: w237 -> [_ w269]
            frame #0 {
            }
            frame #1 {
              n110 = Number To Decimal String(number=w269) -> (decimal integer string=w276:string)  [unwired: 1 in]
              n111 = Format Into String(initial string="waveform_", w276) -> (resulting string=w274:string)  [unwired: 2 in, 1 out]
              n112 = call "Convert to Dynamic Data"("2D Array"=w279) -> ("Dynamic Data Type"=w278:dynamicdata)  [unwired: 3 in]
              n113 = Concatenate Strings(w274, ".txt" ("string")) -> (w273:string)
              n114 = Build Path(base path=w270, name or relative path=w273) -> (appended path=w271:path)
              n115 = call "Write To Measurement File"("Signals"=w278, "error in (no error)"=w268, "Filename"=w271) -> ("error out"=w277:errorcluster)  [unwired: 14 in, 2 out]
            }
          }
        }
      }
      n116 = TCP Close Connection(connection ID=w102, error in (no error)=w103) -> (error out=w104:errorcluster)  [unwired: 1 in, 1 out]
      n117 = stacked-sequence {
        tunnel: w104 -> [w151 _]
        tunnel: [w150 _] -> w89
        tunnel: w112 -> [w149 _]
        tunnel: [w148 _] -> w95
        frame #0 {
          w152 = u16 1 items=["Immediate", "Internal", "External", "Software Trigger Function"] ("Trigger Source (0: Immediate)")
          w153 = u16 0 items=["Edge", "Level"] ("Trigger Mode (0: Edge)")
          # "Probably it could be removed. \nBut I can't probe"
          # "Reset pulse generator tirgger"
          n118 = call "Configure Trigger.vi"("Trigger Source (0: Immediate)"=w152, "error in (no error)"=w151, "Trigger Mode (0: Edge)"=w153, "VISA resource name"=w149) -> ("error out"=w150:errorcluster, "VISA resource name out"=w148:refnum<visa-resource-name>)  [unwired: 6 in]
        }
        frame #1 {
          # "Save data"
          n119 = local write "End 2"(TRUE ("End 2")) -> ()
        }
      }
      n120 = Unbundle By Name(w93) -> ("report out"=w90:refnum<class "NI_report.lvclass">)
      n121 = Bundle By Name(cluster=w93, "report out"=w90, "AWG VISA"=w95, "Oscilloscope  VISA"=w94) -> (w113:T1)
    }
  }
  "Instrument VISA out" <- w18
  n122 = Unbundle By Name(w18) -> ("AWG VISA"=w36:refnum<visa-resource-name>, "Oscilloscope  VISA"=w37:refnum<visa-resource-name>)
  n123 = call "Close.vi"("error in (no error)"=w35, "VISA resource name"=w37) -> ("error out"=w38:errorcluster)  [unwired: 9 in]
  n124 = call "Close.vi"("error in (no error)"=w38, "VISA resource name"=w36) -> ("error out"=→"error out":errorcluster)  [unwired: 9 in]
